vi "DSF.Memory.Pointer.Array.Set Element Size.vi"(8 "error in (no error)":errorcluster, 10 "element size":u64 format="%d bytes", 11 "Array Pointer in":refnum<class "DSF.Memory.Pointer.Array.lvclass">) -> (0 "error out":errorcluster, 3 "Array Pointer out":refnum<class "DSF.Memory.Pointer.Array.lvclass">)   [LabVIEW 2016, in "DSF.Memory.lvlib" / "DSF.Memory.Pointer.Array.lvclass"]
uses:
  DSF.Memory.Pointer.Array.lvclass
  DSF.Memory.Pointer.Array.lvclass/DSF.Memory.Pointer.Array.ctl
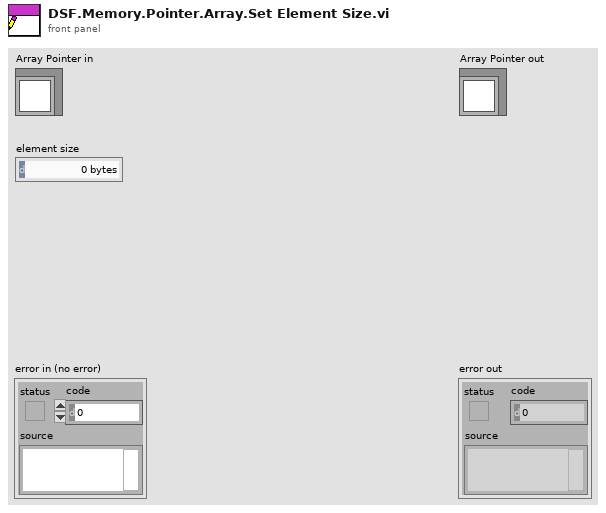
[diagram p1: front panel]
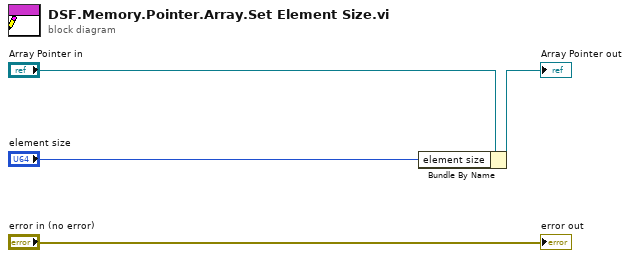
[diagram p0: block diagram]
diagram:
  n1 = Bundle By Name(cluster="Array Pointer in", "element size"="element size") -> (→"Array Pointer out":refnum<class "DSF.Memory.Pointer.Array.lvclass">)
  "error out" <- "error in (no error)"
